vi "FGV_MIDASReply.vi"(7 "Enum":T1, 11 "MIDAS Reply":string) -> (3 "MIDAS Reply":string)   [LabVIEW 2018, in "feGEM DataPacker.lvlib"]
uses:
  Set_And_Get_Enum.ctl
  feGEM DataPacker.lvlib
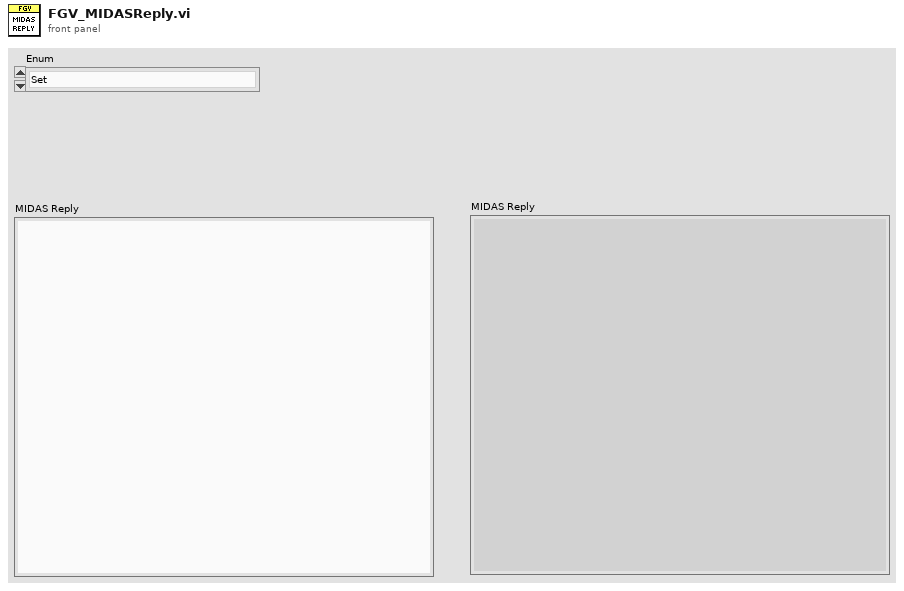
[diagram p1: front panel]
types:
  T1 = typedef "feGEM DataPacker.lvlib/Set_And_Get_Enum.ctl" = enum16{"Set", "Get"}
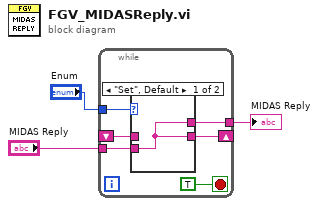
[diagram p0: block diagram]
diagram:
  n1 = while {
    tunnel: "Enum" -> [w9]
    tunnel: [w8] -> w2
    tunnel: "MIDAS Reply" -> [w7]
    shift-right: [w6] -> _
    shift-left: _ -> [w5]
    stop <- TRUE stop-if-true
    n2 = case shown="\"Set\", Default" w9 {
      tunnel: [w10 w11] -> w8
      tunnel: w7 -> [w10 _]
      tunnel: [w10 w11] -> w6
      tunnel: w5 -> [_ w11]
      frame "Set", Default {
      }
      frame "Get" {
      }
    }
  }
  "MIDAS Reply" <- w2
